vi "Destroy.vi"(11 "Hello World Event in":refnum<class "Hello World Event.lvclass">) -> (3 "Hello World Event out":refnum<class "Hello World Event.lvclass">)   [LabVIEW 2021, in "Hello World Event.lvlib" / "Hello World Event.lvclass"]
uses:
  Hello World Event.lvclass
  Hello World Event.lvclass/Hello World Event.ctl
  <vilib>/Nathan Davis/jettl/jettl/Event/Event.lvclass
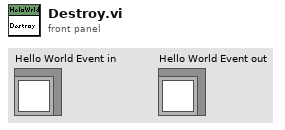
[diagram p1: front panel]
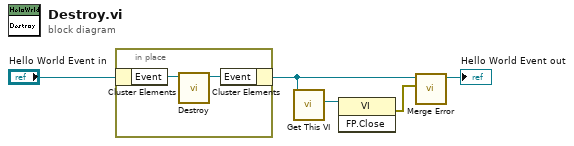
[diagram p0: block diagram]
diagram:
  n1 = in-place {
    n2 = in-place-cluster #1("Hello World Event in") -> ("Event"=w7:refnum<class "Event.lvclass">)
    n3 = call-dynamic "Destroy.vi"("jettl in"=w7) -> ("jettl out"=w6:refnum<class "Event.lvclass">)  [unwired: 10 in]
    n4 = in-place-cluster #1("Event"=w6) -> (w2:refnum<class "Hello World Event.lvclass">)
  }
  n5 = call-dynamic "Get This VI.vi"("Hello World Event in"=w2) -> ("This VI"=w4:refnum<vi>)  [unwired: 10 in]
  n6 = invoke class="VI" method="FP.Close"(reference=w4) -> (error out=w3:errorcluster)  [unwired: 2 in, 2 out]
  n7 = call-dynamic "Merge Error.vi"("Error"=w3, "Hello World Event in"=w2) -> ("Hello World Event out"=→"Hello World Event out":refnum<class "Hello World Event.lvclass">)  [unwired: 9 in]
